vi "Bounds.vi"(1 "XRef":refnum<vi>, 2 "State In":T2) -> (0 "Bounds":cluster{"Width":T1, "Height":T1})   [LabVIEW 2010, in "CData Flatten XNode.xnode"]
doc: "This ability VI is used to tell LabVIEW your current bounds. If you want to update your bounds, you must inform LabVIEW through the UpdateImageAndBounds reply of another ability VI. If you change your bounds, you will also probably want to update your image.\n\nDefault behavior: None.\n\nThis ability does not provide UI and OS messages are not handled."
uses:
  CData Flatten XNode.xnode
  State.ctl
  <vilib>/XNodeSupport/XNodeInt.ctl
  <vilib>/XNodeSupport/NI_XNodeSupport.lvlib
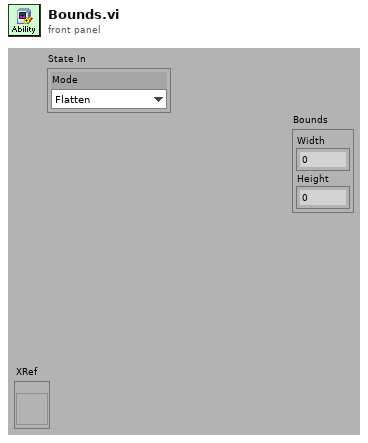
[diagram p1: front panel]
types:
  T1 = typedef "NI_XNodeSupport.lvlib/XNodeInt.ctl" = i32
  T2 = typedef "CData Flatten XNode.xnode/State.ctl" = cluster{"Mode":enum16{"Flatten", "Unflatten"}}
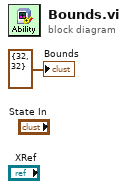
[diagram p0: block diagram]
diagram:
  "Bounds" <- cluster{"Width":T1, "Height":T1} {"Width"=32, "Height"=32} ("Bounds")
